vi "adc_write.vi"(0 "Refnum In":refnum<k20>, 5 "ADC Select":u8(ring) items=["ADC A", "ADC B", "ADC C", "ADC D"], 7 "SPI Addr":u16, 9 "Value":u16(ring) items=["0.0", "0.125", "0.250", "0.375", "0.5", "0.625", "0.75", "0.875"], 11 "error in (no error)":errorcluster) -> (4 "Refnum Out":refnum<k20>, 15 "error out":errorcluster)   [LabVIEW 2015]
uses:
  <vilib>/Utility/error.llb/Error Cluster From Error Code.vi
  <vilib>/rvi/errors/niLvFpgaAdjustHostInterfaceError.vi
  <vilib>/rvi/interface/nirviReadWriteControl/nirviReadWriteControl.xnode
  <vilib>/rvi/interface/Simulation/niFpgaSimulationCallBeginRW.vi
  NiFpgaLv.dll
panel:
  out "Configured?":bool
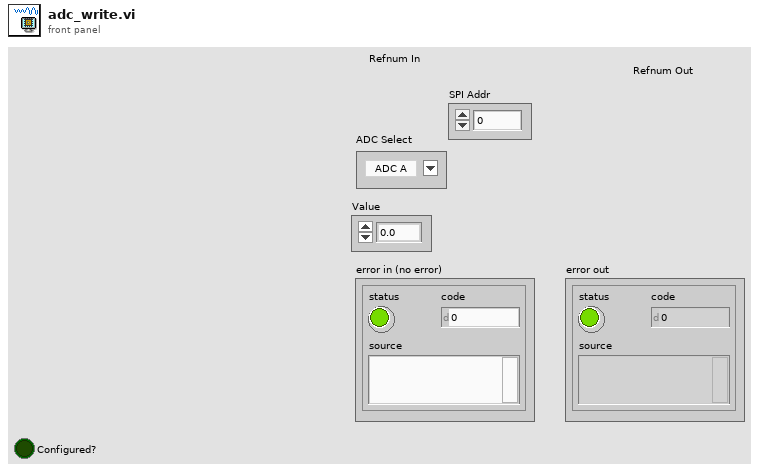
[diagram p1: front panel]
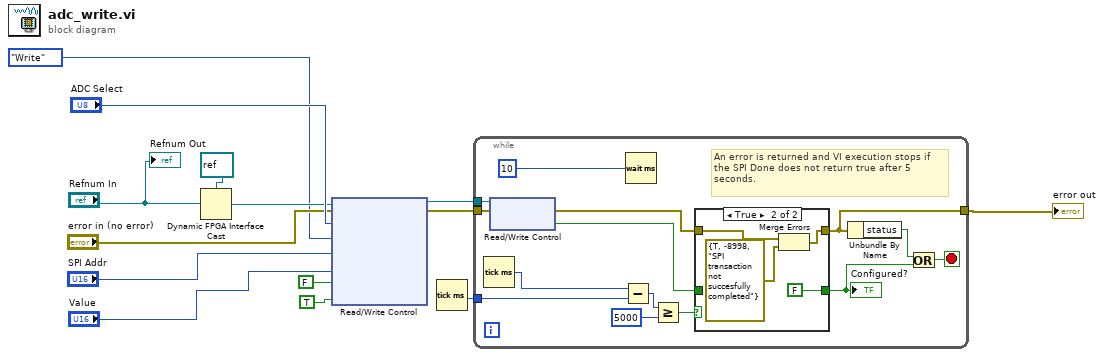
[diagram p0: block diagram]
diagram:
  n1 = Dynamic FPGA Interface Cast(Session In=refnum<k20> refnum ("FPGA VI Reference Out"), Type="Refnum In") -> (Session Out=w7:refnum<k20>)
  n2 = xnode "Read/Write Control"("FPGA VI Reference In"=w7, "error in"="error in (no error)", "SPI ADC Select"="ADC Select", "SPI R/W Select"=enum16{"Read", "Write"}."Write", "SPI Addr"="SPI Addr", "SPI Write Data"="Value", "TGC Enable"=FALSE, "SPI Start"=TRUE ("SpiStart")) -> ("FPGA VI Reference Out"=w10:refnum<k20>, "error out"=w9:errorcluster)
  n3 = Tick Count (ms)() -> (millisecond timer value=w11:u32)
  n4 = while {
    tunnel: w9 -> [w21]
    tunnel: [w25] -> w8
    tunnel: w10 -> [w20]
    tunnel: w11 -> [w16]
    stop <- w23 stop-if-true
    # "An error is returned and VI execution stops if the SPI Done does not return true after 5 seconds."
    n5 = Tick Count (ms)() -> (millisecond timer value=w17:u32)
    n6 = xnode "Read/Write Control"("FPGA VI Reference In"=w20, "error in"=w21) -> ("error out"=w18:errorcluster, "SPI Done"=w19:bool)  [unwired: 1 out]
    n7 = Subtract(x=w17, y=w16) -> (x-y=w15:u32)
    n8 = Wait (ms)(milliseconds to wait=u32 10) -> ()  [unwired: 1 out]
    n9 = Greater Or Equal?(x=w15, y=u32 5000) -> (x >= y?=w26:bool)
    n10 = case shown="True" w26 {
      tunnel: [w30 FALSE ("Configured?")] -> w22
      tunnel: w19 -> [w30 _]
      tunnel: [w29 w33] -> w25
      tunnel: w18 -> [w29 w31]
      frame False {
      }
      frame True {
        n11 = Merge Errors(w31, errorcluster {"status"=TRUE, "code"=-8998, "source"="SPI transaction not succesfully completed"} ("error in")) -> (w33:errorcluster)
      }
    }
    "Configured?" <- w22
    n12 = Unbundle By Name(w25) -> ("status"=w24:bool)
    n13 = Or(x=w24, y=w22) -> (x .or. y?=w23:bool)
  }
  "error out" <- w8
  "Refnum Out" <- "Refnum In"
